vi "CAENHV Init System.vi"(6 "Passwd":string, 7 "UserName":string, 8 "error in (no error)":errorcluster, 9 "Arg":string, 10 "LinkType":i32(ring) items=["TCP/IP"=0, "HS CAENET"=2, "USB 2.0"=3, "CONET Optical Link"=4, "USB VCP"=5], 11 "system":u32(ring) items=["SY1527", "SY2527", "SY4527", "SY5527", "N568", "V65XX", "N1470", "V8100"]) -> (0 "error out":errorcluster, 3 "handle":i32)   [LabVIEW 2014, in "CAENHVWrapper.lvlib"]
doc: "CAENHVLIB_API CAENHVRESULT CAENHV_InitSystem(CAENHV_SYSTEM_TYPE_t system, int LinkType, void *Arg, const char *UserName, const char *Passwd, int *handle);"
uses:
  CAENHVWrapper.lvlib
  CAENHVWrapper.dll
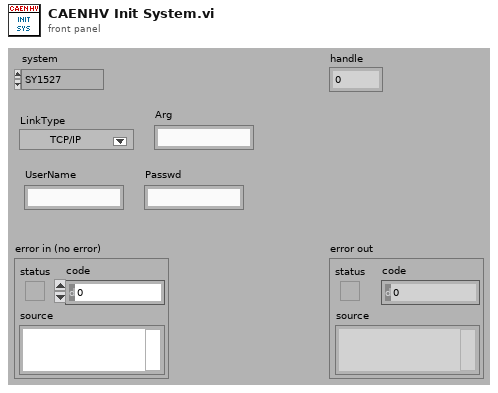
[diagram p1: front panel]
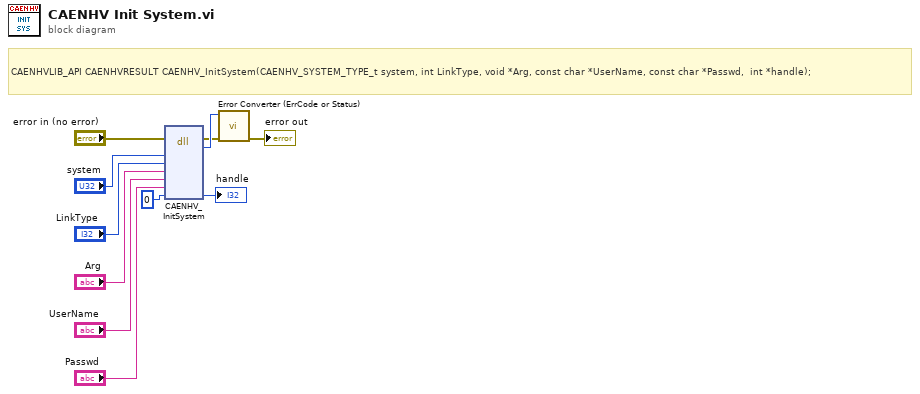
[diagram p0: block diagram]
diagram:
  # "CAENHVLIB_API CAENHVRESULT CAENHV_InitSystem(CAENHV_SYSTEM_TYPE_t system, int LinkType, void *Arg, const char *UserName, const char *Passwd,  int *handle);"
  n1 = dll-call lib="CAENHVWrapper.*" fn="CAENHV_InitSystem"(error in="error in (no error)", "system"="system", "LinkType"="LinkType", "Arg"="Arg", "UserName"="UserName", "Passwd"="Passwd", "handle"=0) -> (error out=w2:errorcluster, "return type"=w3:i32, "handle"=→"handle":i32)  [unwired: 7 in, 1 out]
  n2 = call "Error Converter (ErrCode or Status).vi"("error in (no error)"=w2, "error code"=w3) -> ("error out"=→"error out":errorcluster)  [unwired: 9 in]
